vi "VISA ReadWrite.vi"(5 "Read byte count":u32=1024, 8 "error in (no error)":errorcluster, 9 "write buffer":string, 10 "milliseconds to wait":u32, 11 "VISA Refnum in":refnum<visa-resource-name>="TCPIP0::127.0.0.1::5025::SOCKET") -> (0 "error out":errorcluster, 1 "read buffer":string="\nOK\n-9.1380180522471278e+01,-8.7561871955884968e+01,-9.3857206221490159e+01,-8.6858133994421038e+01,-9.2478674113988177e+01,-9.0923276531138669e+01,-8.5412713079243062e+01,-1.0680557752551536e+02,-9.8139396247310913e+01,-9.5942388317685925e+01,-8.8070150545760754e+01,-8.6010589064907776e+01,-8.1381403758226128e+01,-8.8612193914124816e+01,-8.8234033228500678e+01,-8.6784736973470515e+01,-8.8390475151936997e+01,-9.0166894093978101e+01,-9.3235516052204275e+01,-9.8498375048397122e+01,-8.9926362074673008e+01,-9.3883535338797174e+01,-9.4616326611874769e+01,-9.1184197705494796e+01,-8.2469727001096260e+01,-9.0246555044546454e+01,-8.5790709978521434e+01,-9.1210294324322035e+01,-9.1528412207460946e+01,-9.1774544150860308e+01,-8.6907110149069169e+01,-8.8657427293260227e+01,-8.3588468477941632e+01,-7.9449634296824570e+01,-8.4863492045148632e+01,-7.7255650086811954e+01,-8.0333893002109264e+01,-8.2062899737639611e+01,-8.9239718140047231e+01,-9.2058942343243828e+01,-8.7435414845914735e+01,-9.2380670007406280e+01,-8.6647335", 3 "VISA Refnum out":refnum<visa-resource-name>="TCPIP0::127.0.0.1::5025::SOCKET", 4 "Read return count":u32, 6 "Write return count":u32=21)   [LabVIEW 2010]
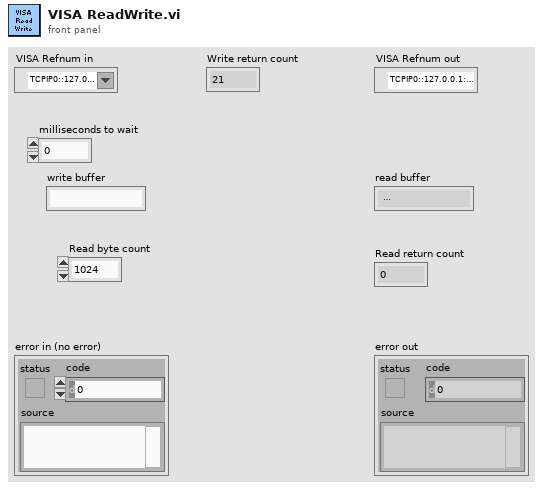
[diagram p1: front panel]
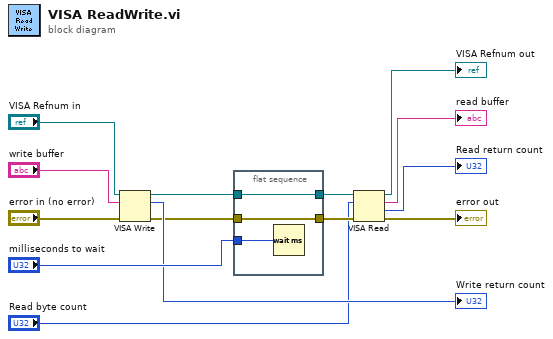
[diagram p0: block diagram]
diagram:
  n1 = VISA Write(VISA resource name="VISA Refnum in", write buffer="write buffer", error in (no error)="error in (no error)") -> (VISA resource name out=w11:refnum<visa-resource-name>, return count=→"Write return count":u32, error out=w1:errorcluster)
  n2 = flat-sequence {
    tunnel: w1 -> [w17]
    tunnel: [w17] -> w9
    tunnel: [w16] -> w10
    tunnel: w11 -> [w16]
    tunnel: "milliseconds to wait" -> [w15]
    frame #0 {
      n3 = Wait (ms)(milliseconds to wait=w15) -> ()  [unwired: 1 out]
    }
  }
  n4 = VISA Read(VISA resource name=w10, byte count="Read byte count", error in (no error)=w9) -> (VISA resource name out=→"VISA Refnum out":refnum<visa-resource-name>, read buffer=→"read buffer":string, return count=→"Read return count":u32, error out=→"error out":errorcluster)
